vi "Make from Project.vi"(8 "error in (no error)":errorcluster, 10 "Project Path":path) -> (0 "error out":errorcluster, 3 "LUnit Test Suite V2 Out":refnum<class "LUnit Test Suite V2.lvclass">)   [LabVIEW 2020, in "LUnit Test Suite V2.lvclass"]
uses:
  LUnit Test Suite V2.lvclass
  C:/Git/astemes-lunit/source/Rewrite Project/Run/Runnable.lvclass
  LUnit Test Case/LUnit Test Case V2.lvclass
  LUnit Test Suite V2.lvclass/LUnit Test Suite V2.ctl
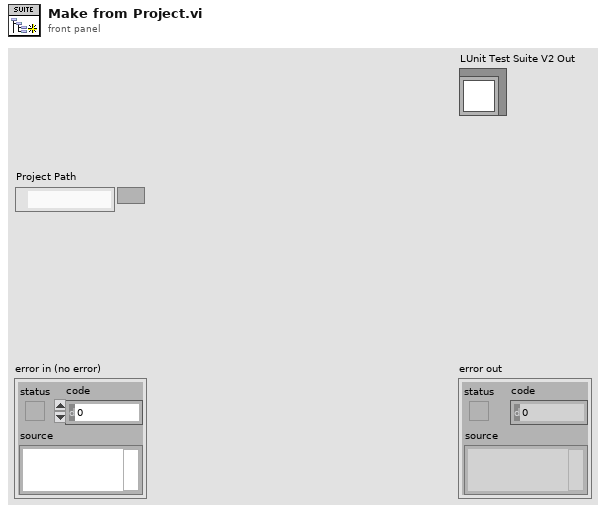
[diagram p1: front panel]
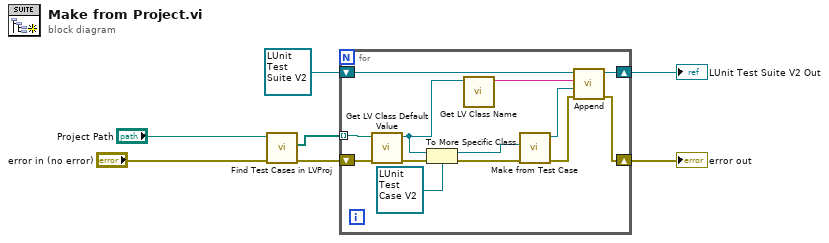
[diagram p0: block diagram]
diagram:
  n1 = call "Find Test Cases in LVProj.vi"("error in (no error)"="error in (no error)", "Project Path"="Project Path") -> ("error out"=w5:errorcluster, "Test Class paths"=w6:path[])  [unwired: 8 in]
  n2 = for {
    tunnel: w6 -> [w10] mode=indexing
    shift-right: [w18] -> w1
    shift-left: refnum<class "LUnit Test Suite V2.lvclass"> refnum ("LUnit Test Suite V2 in") -> [w19]
    shift-right: [w15] -> w3
    shift-left: w5 -> [w20]
    n3 = call <vilib>:"Get LV Class Default Value.vi"("error in (no error)"=w20, "class path"=w10) -> ("error out"=w17:errorcluster, "object"=w9:refnum<class>)  [unwired: 8 in]
    n4 = To More Specific Class(target class=refnum<class "LUnit Test Case V2.lvclass"> refnum ("LUnit Test Case V2.lvclass"), reference=w9, error in=w17) -> (specific class reference=w12:refnum<class "LUnit Test Case V2.lvclass">, error out=w14:errorcluster)
    n5 = call <vilib>:"Get LV Class Name.vi"("object"=w9) -> ("class name"=w8:string)  [unwired: 9 in, 1 out]
    n6 = call "Make from Test Case.vi"("error in (no error)"=w14, "LUnit Test Case"=w12) -> ("error out"=w13:errorcluster, "LUnit Test Suite V2 out"=w11:refnum<class "LUnit Test Suite V2.lvclass">)  [unwired: 8 in]
    n7 = call "Append.vi"("error in (no error)"=w13, "Runnable"=w11, "Name"=w8, "LUnit Test Suite V2 in"=w19) -> ("error out"=w15:errorcluster, "LUnit Test Suite V2 out"=w18:refnum<class "LUnit Test Suite V2.lvclass">)  [unwired: 6 in]
  }
  "error out" <- w3
  "LUnit Test Suite V2 Out" <- w1
